vi "CanSetParameterIntegerValue.vi"(6 "ParameterValue":i64, 8 "error in (no error)":errorcluster, 10 "PicamParameter":T1 items=["ExposureTime"=33685527, "ShutterTimingMode"=50593816, "ShutterOpeningDelay"=33685550, "ShutterClosingDelay"=33685529, "ShutterDelayResolution"=50462767, "InternalShutterType"=17039499, "InternalShutterStatus"=17039513, "ExternalShutterType"=17039512, "ExternalShutterStatus"=17039514, "ActiveShutter"=50593947, "InactiveShutterTimingModeResult"=17039516, "GatingMode"=50593885, "RepetitiveGate"=84344926, "SequentialStartingGate"=84344927, "SequentialEndingGate"=84344928, "SequentialGateStepCount"=33947745, "SequentialGateStepIterations"=33947746, "DifStartingGate"=84344934, "DifEndingGate"=84344935, "EnableIntensifier"=50528342, "IntensifierStatus"=17039447, "IntensifierGain"=33620056, "EMIccdGainControlMode"=50593915, "EMIccdGain"=33620092, "PhosphorDecayDelay"=33685593, "PhosphorDecayDelayResolution"=50462810, "BracketGating"=50528356, "IntensifierOptions"=17039461, "EnableModulation"=50528367, "ModulationDuration"=33685622, "ModulationFrequency"=33685616, "RepetitiveModulationPhase"=33685617, "SequentialStartingModulationPhase"=33685618, "SequentialEndingModulationPhase"=33685619, "CustomModulationSequence"=134742135, "PhotocathodeSensitivity"=17039467, "GatingSpeed"=17039468, "PhosphorType"=17039469, "IntensifierDiameter"=16908398, "AdcSpeed"=50462753, "AdcBitDepth"=50397218, "AdcAnalogGain"=50593827, "AdcQuality"=50593828, "AdcEMGain"=33620021, "CorrectPixelBias"=50528362, "TriggerSource"=50593871, "TriggerResponse"=50593822, "TriggerDetermination"=50593823, "TriggerFrequency"=33685584, "TriggerTermination"=50593873, "TriggerCoupling"=50593874, "TriggerThreshold"=33685587, "TriggerDelay"=33685668, "OutputSignal"=50593824, "InvertOutputSignal"=50528308, "OutputSignal2"=50593942, "InvertOutputSignal2"=50528407, "EnableAuxOutput"=50528417, "AuxOutput"=84344923, "EnableSyncMaster"=50528340, "SyncMaster2Delay"=33685589, "EnableModulationOutputSignal"=50528372, "ModulationOutputSignalFrequency"=33685621, "ModulationOutputSignalAmplitude"=33685624, "AnticipateTrigger"=50528387, "DelayFromPreTrigger"=33685636, "ReadoutControlMode"=50593818, "ReadoutTimeCalculation"=16908315, "ReadoutPortCount"=50397212, "ReadoutOrientation"=17039414, "KineticsWindowHeight"=33620024, "SeNsRWindowHeight"=33620131, "VerticalShiftRate"=50462733, "Accumulations"=33947740, "EnableNondestructiveReadout"=50528384, "NondestructiveReadoutPeriod"=33685633, "Rois"=67436581, "NormalizeOrientation"=50528295, "DisableDataFormatting"=50528311, "ReadoutCount"=33947688, "ExactReadoutCountMaximum"=17170509, "PhotonDetectionMode"=50593917, "PhotonDetectionThreshold"=33685630, "PixelFormat"=50593833, "FrameSize"=16842794, "FrameStride"=16842795, "FramesPerReadout"=16842796, "ReadoutStride"=16842797, "PixelBitDepth"=16842800, "ReadoutRateCalculation"=16908338, "OnlineReadoutRateCalculation"=16908387, "FrameRateCalculation"=16908339, "Orientation"=17039398, "TimeStamps"=50593860, "TimeStampResolution"=50724933, "TimeStampBitDepth"=50397254, "TrackFrames"=50528327, "FrameTrackingBitDepth"=50397256, "GateTracking"=50593896, "GateTrackingBitDepth"=50397289, "ModulationTracking"=50593913, "ModulationTrackingBitDepth"=50397306, "SensorType"=17039417, "CcdCharacteristics"=17039418, "SensorActiveWidth"=16842811, "SensorActiveHeight"=16842812, "SensorActiveExtendedHeight"=16842911, "SensorActiveLeftMargin"=16842813, "SensorActiveTopMargin"=16842814, "SensorActiveRightMargin"=16842815, "SensorActiveBottomMargin"=16842816, "SensorMaskedHeight"=16842817, "SensorMaskedTopMargin"=16842818, "SensorMaskedBottomMargin"=16842819, "SensorSecondaryMaskedHeight"=16842801, "SensorSecondaryActiveHeight"=16842826, "PixelWidth"=16908297, "PixelHeight"=16908298, "PixelGapWidth"=16908299, "PixelGapHeight"=16908300, "ApplicableStarDefectMapID"=16842918, "ActiveWidth"=33619969, "ActiveHeight"=33619970, "ActiveExtendedHeight"=33620128, "ActiveLeftMargin"=33619971, "ActiveTopMargin"=33619972, "ActiveRightMargin"=33619973, "ActiveBottomMargin"=33619974, "MaskedHeight"=33619975, "MaskedTopMargin"=33619976, "MaskedBottomMargin"=33620041, "SecondaryMaskedHeight"=33620043, "SecondaryActiveHeight"=33620044, "CleanSectionFinalHeight"=33619985, "CleanSectionFinalHeightCount"=33619986, "CleanSerialRegister"=50528275, "CleanCycleCount"=33619988, "CleanCycleHeight"=33619989, "CleanBeforeExposure"=50528334, "CleanUntilTrigger"=50528278, "StopCleaningOnPreTrigger"=50528386, "SensorTemperatureSetPoint"=33685518, "SensorTemperatureReading"=16908303, "SensorTemperatureStatus"=17039376, "DisableCoolingFan"=50528285, "CoolingFanStatus"=17039522, "EnableSensorWindowHeater"=50528383, "VacuumStatus"=17039525, "CenterWavelengthSetPoint"=33685644, "CenterWavelengthReading"=16908429, "CenterWavelengthStatus"=17039509, "GratingType"=17039502, "GratingCoating"=17039503, "GratingGrooveDensity"=16908432, "GratingBlazingWavelength"=16908433, "FocalLength"=16908434, "InclusionAngle"=16908435, "SensorAngle"=16908436, "LightSource"=50593925, "LightSourceStatus"=17039494, "Age"=16908423, "LifeExpectancy"=16908424, "LaserOutputMode"=50593929, "LaserPower"=33685642, "LaserStatus"=17039517, "InputTriggerStatus"=17039518], 11 "PicamHandle in":u64) -> (0 "error out":errorcluster, 2 "Valid":bool, 3 "PicamHandle out":u64)   [LabVIEW 2019, in "PICam.lvlib"]
uses:
  PICam.lvlib
  types/PicamParameter.ctl
  Ctrls/PicamErrors.ctl
  Picam64.dll
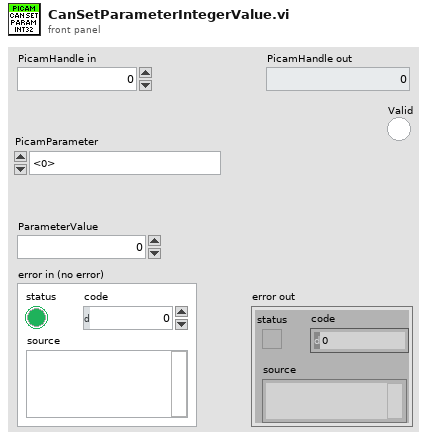
[diagram p1: front panel]
types:
  T1 = typedef "PICam.lvlib/PicamParameter.ctl" = i32
  T2 = typedef "PICam.lvlib/PicamErrors.ctl" = i32
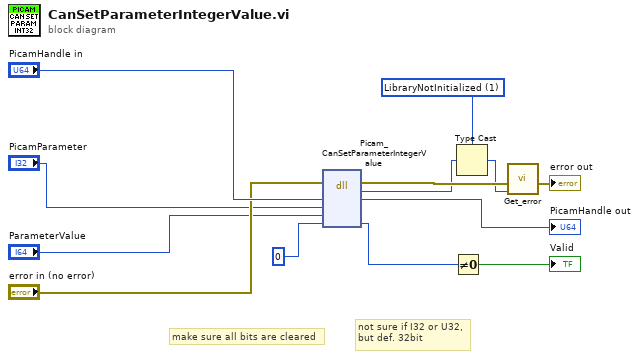
[diagram p0: block diagram]
diagram:
  w11 = T2 1 items=["LibraryNotInitialized"=1, "InvalidParameterValue"=2, "UnexpectedNullPointer"=3, "UnexpectedError"=4, "LibraryAlreadyInitialized"=5, "InvalidDemoModel"=6, "CameraAlreadyOpened"=7, "InvalidCameraID"=8, "InvalidHandle"=9, "ParameterValueIsReadOnly"=10, "ParameterHasInvalidValueType"=11, "ParameterDoesNotExist"=12, "ParameterHasInvalidConstraintType"=13, "ParameterValueIsIrrelevant"=14, "DeviceCommunicationFailed"=15, "InvalidEnumeratedType"=16, "EnumerationValueNotDefined"=17, "NotDiscoveringCameras"=18, "AlreadyDiscoveringCameras"=19, "AcquisitionInProgress"=20, "InvalidDemoSerialNumber"=21, "DemoAlreadyConnected"=22, "DeviceDisconnected"=23, "DeviceOpenElsewhere"=24, "ParameterIsNotOnlineable"=25, "ParameterIsNotReadable"=26, "AcquisitionNotInProgress"=27, "InvalidParameterValues"=28, "ParametersNotCommitted"=29, "InvalidAcquisitionBuffer"=30, "InsufficientMemory"=31, "TimeOutOccurred"=32, "AcquisitionUpdatedHandlerRegistered"=33, "NoCamerasAvailable"=34, "InvalidPointer"=35, "InvalidReadoutCount"=36, "InvalidReadoutTimeOut"=37, "InvalidConstraintCategory"=38, "InvalidCount"=39, "DemoNotSupported"=40, "NondestructiveReadoutEnabled"=41, "InvalidOperation"=42, "OperationCanceled"=43, "InvalidAcquisitionState"=44, "NoAccessoriesAvailable"=45, "AccessoryAlreadyOpened"=46, "InvalidAccessoryID"=47, "NotDiscoveringAccessories"=48, "AlreadyDiscoveringAccessories"=49, "ParameterIsNotWaitableStatus"=50, "InvalidWaitableStatusParameterTimeOut"=51, "ShutterOverheated"=52, "CameraFaulted"=53, "CenterWavelengthFaulted"=54] ("PICam_Error")
  # "not sure if I32 or U32,\nbut def. 32bit"
  # "make sure all bits are cleared"
  n1 = dll-call lib="Picam*.*" fn="Picam_CanSetParameterIntegerValue"(error in="error in (no error)", "PicamHandle"="PicamHandle in", "PicamParameter"="PicamParameter", "ParameterValue"="ParameterValue", "Valid"=0) -> (error out=w13:errorcluster, "error"=w5:i64, "PicamHandle"=→"PicamHandle out":i64, "Valid"=w3:i32)  [unwired: 4 in, 1 out]
  n2 = Not Equal To 0?(x=w3) -> (x != 0?=→"Valid":bool)
  n3 = Type Cast(type=w11, x=w5) -> (*(type *) &x=w12:T2)
  n4 = call "Get_error.vi"("PICam_Error"=w12, "error in (no error)"=w13) -> ("error out"=→"error out":errorcluster)  [unwired: 9 in]
